vi "Read APIs.vi"(8 "error in (no error)":errorcluster, 11 "CSM-Helper in":refnum<class "CSM-Helper.lvclass">) -> (0 "error out":errorcluster, 2 "Value":string[](array[string]), 3 "CSM-Helper out":refnum<class "CSM-Helper.lvclass">)   [LabVIEW 2020, in "CSM-Helper.lvclass"]
uses:
  CSM-Helper.lvclass
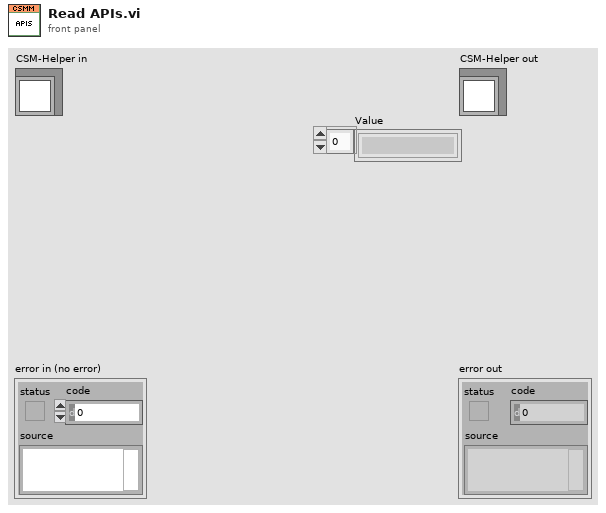
[diagram p1: front panel]
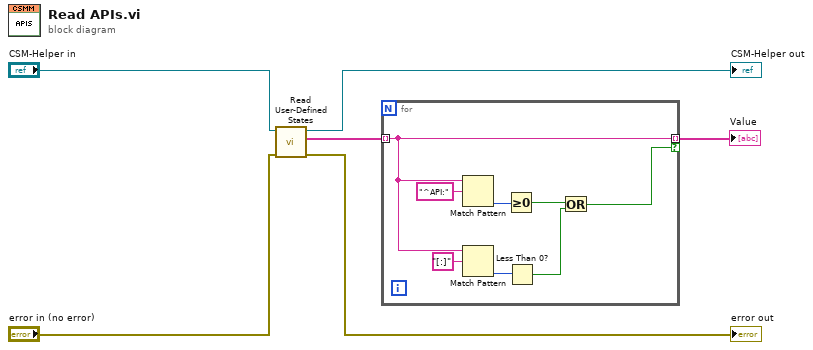
[diagram p0: block diagram]
diagram:
  n1 = call "Read User-Defined States.vi"("error in (no error)"="error in (no error)", "CSM-Helper in"="CSM-Helper in") -> ("error out"=→"error out":errorcluster, "Array"=w2:string[], "CSM-Helper out"=→"CSM-Helper out":refnum<class "CSM-Helper.lvclass">)  [unwired: 7 in]
  n2 = for {
    tunnel: w2 -> [w10] mode=indexing
    tunnel: [w10] -> w1 mode=indexing if=w7
    n3 = Match Pattern(string=w10, regular expression="^API:") -> (offset past match=w12:i32)  [unwired: 1 in, 3 out]
    n4 = Match Pattern(string=w10, regular expression="[:]") -> (offset past match=w11:i32)  [unwired: 1 in, 3 out]
    n5 = Greater Or Equal To 0?(x=w12) -> (x >= 0?=w9:bool)
    n6 = Less Than 0?(x=w11) -> (x < 0?=w8:bool)
    n7 = Or(x=w9, y=w8) -> (x .or. y?=w7:bool)
  }
  "Value" <- w1
